vi "Connect and query.vi"(8 "error in (no error)":errorcluster, 11 "COM params":T1 {"COM params"."stop bits" items=["1.0"=10, "1.5"=15, "2.0"=20]; "COM params"."flow control" items=["None", "XON/XOFF", "RTS/CTS", "XON/XOFF & RTS/CTS", "DTR/DSR", "XON/XOFF & DTR/DSR"]}) -> (0 "error out":errorcluster, 2 "Connected?":bool, 3 "VISA Refnum":refnum<visa-resource-name>)   [LabVIEW 2020, in "Arduino stepper.lvlib"]
uses:
  Arduino stepper.lvlib
  Connect Argument--cluster.ctl
  COM params--typedef.ctl
  <vilib>/Instr/_visa.llb/VISA Configure Serial Port (Instr).vi
panel:
  out "read buffer":string
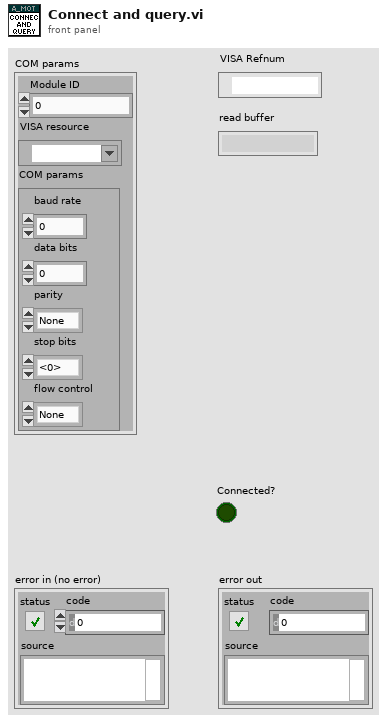
[diagram p1: front panel]
types:
  T1 = typedef "Arduino stepper.lvlib/Connect Argument--cluster.ctl" = cluster{"Module ID":i32, "VISA resource":refnum<visa-resource-name>, "COM params":T2}
  T2 = typedef "Arduino stepper.lvlib/COM params--typedef.ctl" = cluster{"baud rate":u32, "data bits":u16, "parity":enum16{"None", "Odd", "Even", "Mark", "Space"}, "stop bits":u16, "flow control":u16}
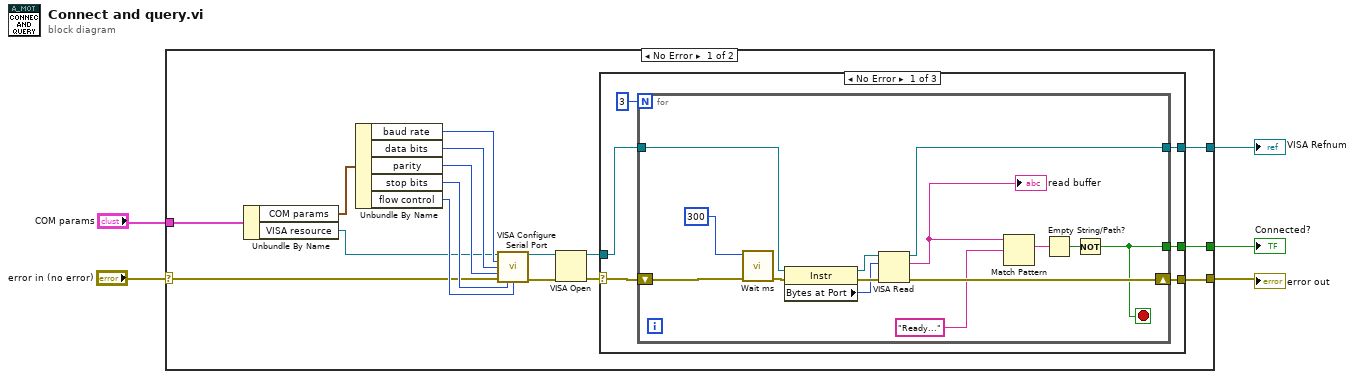
[diagram p0: block diagram]
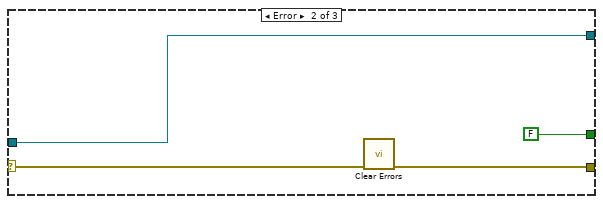
[diagram p2: hidden frame]
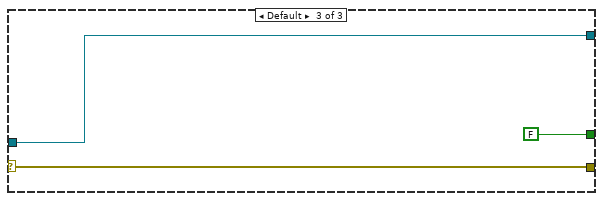
[diagram p3: hidden frame]
diagram:
  n1 = case shown="No Error" "error in (no error)" {
    selector: "error in (no error)" -> [w14 w49]
    tunnel: [w11 _] -> w5
    tunnel: [w12 w49] -> w4
    tunnel: "COM params" -> [w13 _]
    tunnel: [w10 _] -> w1
    frame No Error {
      n2 = Unbundle By Name(w13) -> ("COM params"=w16:T2, "VISA resource"=w15:refnum<visa-resource-name>)
      n3 = Unbundle By Name(w16) -> ("baud rate"=w17:u32, "data bits"=w18:u16, "parity"=w19:enum16{"None", "Odd", "Even", "Mark", "Space"}, "stop bits"=w20:u16, "flow control"=w21:u16)
      n4 = call-poly "VISA Configure Serial Port"("VISA resource name"=w15, "baud rate (9600)"=w17, "data bits (8)"=w18, "parity (0:none)"=w19, "error in (no error)"=w14, "stop bits (10: 1 bit)"=w20, "flow control (0:none)"=w21) -> ("VISA resource name out"=w9:refnum<visa-resource-name>, "error out"=w7:errorcluster)  [unwired: 7 in]
      n5 = VISA Open(error in (no error)=w7, VISA resource name=w9) -> (VISA resource name=w8:refnum<visa-resource-name>, error out=w6:errorcluster)  [unwired: 3 in]
      n6 = case shown="No Error" w6 {
        selector: w6 -> [w23 w45 w48]
        tunnel: [w26 w43 w48] -> w12
        tunnel: [w25 w44 w47] -> w11
        tunnel: [w24 FALSE FALSE] -> w10
        tunnel: w8 -> [w27 w44 w47]
        frame No Error {
          n7 = for {
            N: 3 -> [_]
            tunnel: [w28] -> w24
            shift-right: [w36] -> w26
            shift-left: w23 -> [w30]
            tunnel: w27 -> [w37]
            tunnel: [w34] -> w25
            stop <- w28 stop-if-true
            n8 = call "Wait ms.vi"("error in (no error)"=w30, "milliseconds to wait"=u32 300) -> ("error out"=w40:errorcluster)  [unwired: 9 in]
            n9 = property class="Instr"(reference=w37, error in=w40) -> (reference out=w38:refnum<visa-resource-name>, error out=w41:errorcluster, "Bytes at Port"=w39:u32)
            n10 = VISA Read(VISA resource name=w38, byte count=w39, error in (no error)=w41) -> (VISA resource name out=w34:refnum<visa-resource-name>, read buffer=w29:string, error out=w36:errorcluster)  [unwired: 1 out]
            "read buffer" <- w29
            n11 = Match Pattern(string=w29, regular expression="Ready..." ("x")) -> (match substring=w32:string)  [unwired: 1 in, 3 out]
            n12 = Empty String/Path?(string/path=w32) -> (empty?=w31:bool)
            n13 = Not(x=w31) -> (.not. x?=w28:bool)
          }
        }
        frame Error {
          n14 = call <vilib>:"Clear Errors.vi"("error in (no error)"=w45) -> ("error out"=w43:errorcluster)  [unwired: 5 in, 1 out]
        }
        frame Default {
        }
      }
    }
    frame Error {
    }
  }
  "VISA Refnum" <- w5
  "error out" <- w4
  "Connected?" <- w1
